vi "TC to PGSQL.vi"(0 "Calibration":refnum<vi>[](array[refnum]), 1 "AVS names":T1, 2 "R":dbl[](array[numeric]), 3 "T":dbl[](array[numeric]), 4 "I":dbl[](array[numeric])) -> ()   [LabVIEW 2019, in "FP-TC-Shared.lvclass"]
uses:
  FP-TC-Shared.lvclass
  FP-TC-Shared.lvclass/FP-TC-Shared.ctl
  <userlib>/LevyLab/LV-Data/LV-Data.PG/LV-Data.PGSQL.lvclass
  <userlib>/LevyLab/LV-Data/LV-Data.PG/API/Write Variable (one-row).vi
panel:
  out "error out":errorcluster
  in  "error in (no error)":errorcluster
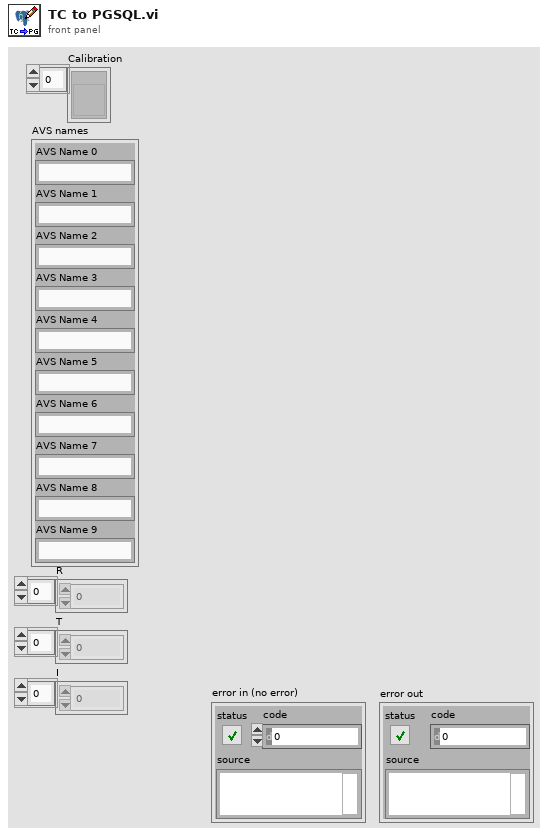
[diagram p1: front panel]
types:
  T1 = cluster{"AVS Name 0":string, "AVS Name 1":string, "AVS Name 2":string, "AVS Name 3":string, "AVS Name 4":string, "AVS Name 5":string, "AVS Name 6":string, "AVS Name 7":string, "AVS Name 8":string, "AVS Name 9":string}
  T2 = typedef "FP-TC-Shared.lvclass/LC Type--Enum.ctl" = enum16{"CF.TC", "CF.TC.Z", "CF.FP", "MNK.TC", "MNK.TC.Z", "MNK.FP"}
  T3 = cluster{dbl[], "delimited string":string, "delimited string":string}
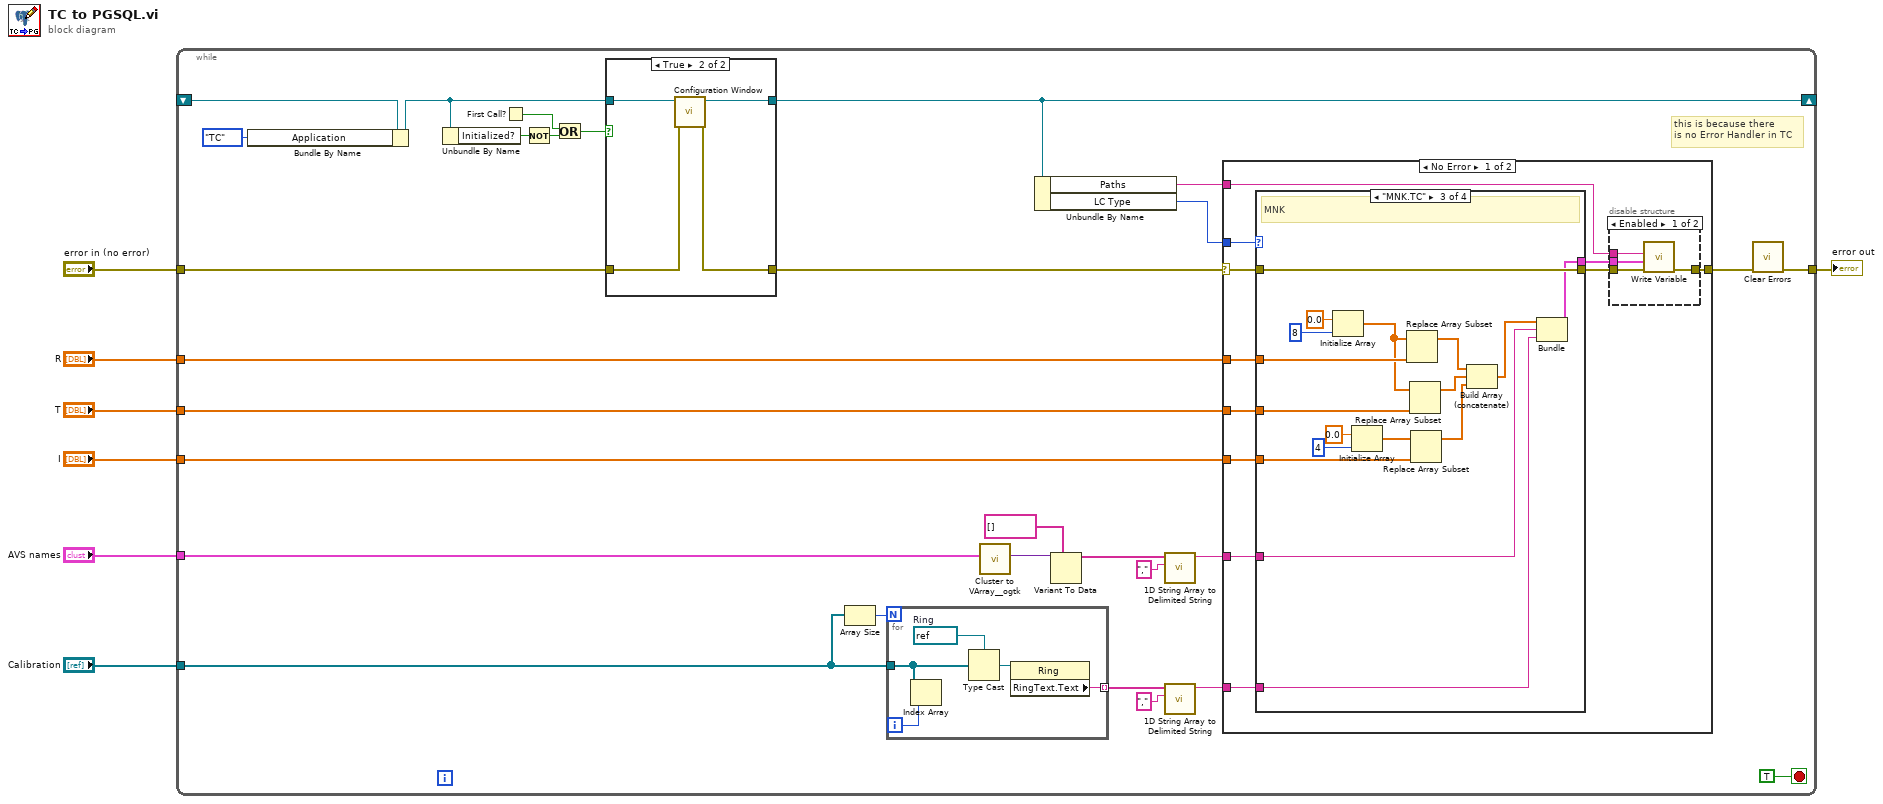
[diagram p0: block diagram]
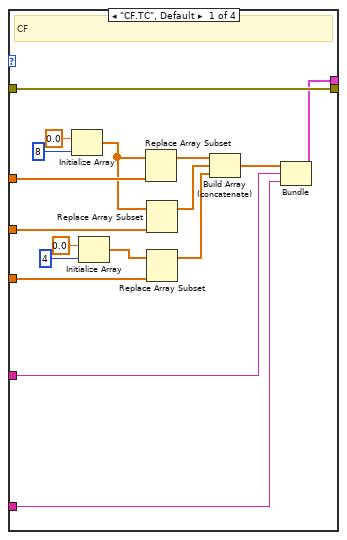
[diagram p4: hidden frame]
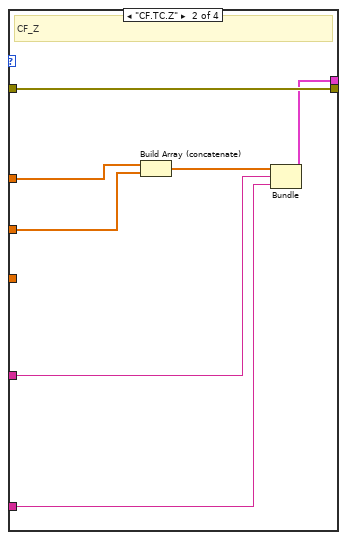
[diagram p5: hidden frame]
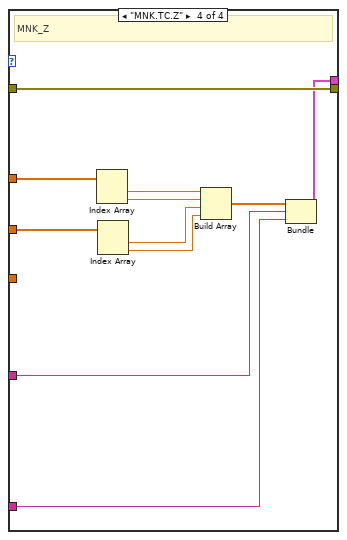
[diagram p6: hidden frame]
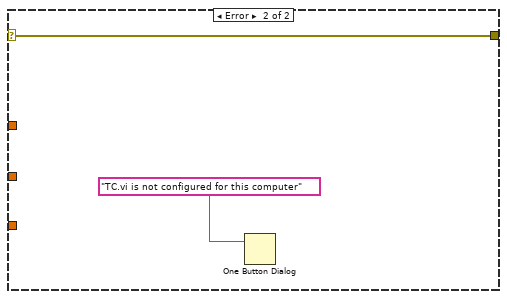
[diagram p7: hidden frame]
diagram:
  n1 = while {
    tunnel: "AVS names" -> [w17]
    tunnel: "I" -> [w34]
    tunnel: "T" -> [w33]
    tunnel: "R" -> [w32]
    tunnel: "Calibration" -> [w31]
    tunnel: "error in (no error)" -> [w23]
    tunnel: [w35] -> w6
    shift-right: [w25] -> _
    shift-left: _ -> [w9]
    stop <- TRUE stop-if-true
    # "this is because there\nis no Error Handler in TC"
    n2 = Bundle By Name(cluster=w9, "Application"=enum16{"TC", "FP"}."TC" ("Configuration.Application")) -> (w8:refnum<class "FP-TC-Shared.lvclass">)
    n3 = Unbundle By Name(w8) -> ("Initialized?"=w28:bool)
    n4 = First Call?() -> (First Call?: T/F=w26:bool)
    n5 = Not(x=w28) -> (.not. x?=w27:bool)
    n6 = Or(x=w26, y=w27) -> (x .or. y?=w29:bool)
    n7 = case shown="True" w29 {
      tunnel: [w38 w41] -> w25
      tunnel: w8 -> [w38 w42]
      tunnel: [w37 w39] -> w24
      tunnel: w23 -> [w37 w40]
      frame False {
      }
      frame True {
        n8 = call-dynamic "Configuration Window.vi"("error in (no error)"=w40, "FP-TC-Shared"=w42) -> ("error out"=w39:errorcluster, "FP-TC-Shared out"=w41:refnum<class "FP-TC-Shared.lvclass">)  [unwired: 8 in]
      }
    }
    n9 = Array Size(array=w31) -> (size(s)=w36:i32)
    n10 = for {
      N: w36 -> [_]
      tunnel: w31 -> [w44]
      tunnel: [w45] -> w22 mode=indexing
      i -> [w43]
      w47 = refnum<vi> refnum  # Ring
      n11 = Index Array(array=w44, index=w43) -> ()  [unwired: 1 out]
      n12 = Type Cast(type=w47, x=w44) -> (*(type *) &x=w46:refnum<vi>)
      n13 = property class="Ring"(reference=w46) -> ("RingText.Text"=w45:string)  [unwired: 1 in, 2 out]
    }
    n14 = call <userlib>:"Cluster to VArray__ogtk.vi"("Cluster"=w17) -> ("VArray"=w16:variant)  [unwired: 9 in, 1 out]
    n15 = Unbundle By Name(w25) -> ("Paths"=w13:string, "LC Type"=w11:T2)
    n16 = Variant To Data(type=string[] [], Variant=w16) -> (data=w15:string[])  [unwired: 1 in, 1 out]
    n17 = call <vilib>:"1D String Array to Delimited String.vi"("delimiter"=",", "string array"=w15) -> ("delimited string"=w18:string)  [unwired: 9 in]
    n18 = call <vilib>:"1D String Array to Delimited String.vi"("delimiter"=",", "string array"=w22) -> ("delimited string"=w20:string)  [unwired: 9 in]
    n19 = case shown="No Error" w24 {
      selector: w24 -> [w52 w115]
      tunnel: w18 -> [w58 _]
      tunnel: w20 -> [w57 _]
      tunnel: w11 -> [w56 _]
      tunnel: w32 -> [w55 _]
      tunnel: w33 -> [w54 _]
      tunnel: w34 -> [w53 _]
      tunnel: w13 -> [w48 _]
      tunnel: [w50 w115] -> w12
      frame No Error {
        n20 = case shown="\"MNK.TC\"" w56 {
          tunnel: w55 -> [w69 w86 w95 w110]
          tunnel: w54 -> [w67 w80 w94 w109]
          tunnel: w53 -> [w70 _ w93 _]
          tunnel: w58 -> [w65 w83 w89 w107]
          tunnel: w57 -> [w66 w82 w88 w106]
          tunnel: w52 -> [w79 w85 w103 w111]
          tunnel: [w79 w85 w103 w111] -> w51
          tunnel: [w63 w81 w87 w105] -> w49
          frame "CF.TC", Default {
            # "CF"
            n21 = Initialize Array(0.0 ("element"), 8 ("dimension size")) -> (w68:dbl[])
            n22 = Initialize Array(0.0 ("element"), 4 ("dimension size")) -> (w72:dbl[])
            n23 = Replace Array Subset(array=w68, new element=w69) -> (w76:dbl[])  [unwired: 1 in]
            n24 = Replace Array Subset(array=w68, new element=w67) -> (w75:dbl[])  [unwired: 1 in]
            n25 = Replace Array Subset(array=w72, new element=w70) -> (w71:dbl[])  [unwired: 1 in]
            n26 = Build Array (concatenate)(w76, w75, w71) -> (w64:dbl[])
            n27 = Bundle(w64, "delimited string"=w65, "delimited string"=w66) -> (w63:T3)  [unwired: 1 in]
          }
          frame "CF.TC.Z" {
            # "CF_Z"
            n28 = Build Array (concatenate)(w86, w80) -> (w84:dbl[])
            n29 = Bundle(w84, "delimited string"=w83, "delimited string"=w82) -> (w81:T3)  [unwired: 1 in]
          }
          frame "MNK.TC" {
            # "MNK"
            n30 = Initialize Array(0.0 ("element"), 8 ("dimension size")) -> (w91:dbl[])
            n31 = Initialize Array(0.0 ("element"), 4 ("dimension size")) -> (w97:dbl[])
            n32 = Replace Array Subset(array=w91, new element=w95) -> (w101:dbl[])  [unwired: 1 in]
            n33 = Replace Array Subset(array=w91, new element=w94) -> (w100:dbl[])  [unwired: 1 in]
            n34 = Replace Array Subset(array=w97, new element=w93) -> (w96:dbl[])  [unwired: 1 in]
            n35 = Build Array (concatenate)(w101, w100, w96) -> (w90:dbl[])
            n36 = Bundle(w90, "delimited string"=w89, "delimited string"=w88) -> (w87:T3)  [unwired: 1 in]
          }
          frame "MNK.TC.Z" {
            # "MNK_Z"
            n37 = Index Array(array=w110) -> (element #1=w114:dbl, element #2=w113:dbl)  [unwired: 2 in]
            n38 = Index Array(array=w109) -> (element #1=w104:dbl, element #2=w112:dbl)  [unwired: 2 in]
            n39 = Build Array(w114, w113, w104, w112) -> (w108:dbl[])
            n40 = Bundle(w108, "delimited string"=w107, "delimited string"=w106) -> (w105:T3)  [unwired: 1 in]
          }
        }
        n41 = disable-structure shown="Enabled" {
          disable-tunnel: w51 -> [w62 _]
          disable-tunnel: [w61 _] -> w50
          disable-tunnel: w49 -> [w60 _]
          disable-tunnel: w48 -> [w59 _]
          frame Enabled {
            n42 = call-poly <userlib>:"Write Variable.vi"("error in (no error)"=w62, "Data"=w60, "variable"=w59) -> ("error out"=w61:errorcluster)  [unwired: 5 in, 3 out]
          }
          frame Disabled {
          }
        }
      }
      frame Error {
        n43 = One Button Dialog(message="TC.vi is not configured for this computer" ("URL")) -> ()  [unwired: 1 in, 1 out]
      }
    }
    n44 = call <vilib>:"Clear Errors.vi"("error in (no error)"=w12) -> ("error out"=w35:errorcluster)  [unwired: 5 in, 1 out]
  }
  "error out" <- w6
